vi "Initialize-buffers.vi"(8 "error in (no error)":errorcluster, 11 "Data ref. in":refnum<data-value>) -> (0 "error out":errorcluster, 3 "Data ref.":refnum<data-value>)   [LabVIEW 2013, in "CameraVision.lvlib" / "CV-Main.lvclass"]
uses:
  CV-Main.lvclass
  Buffers/CV-Buffers.lvclass
  CV-Main.lvclass/CV-Main.ctl
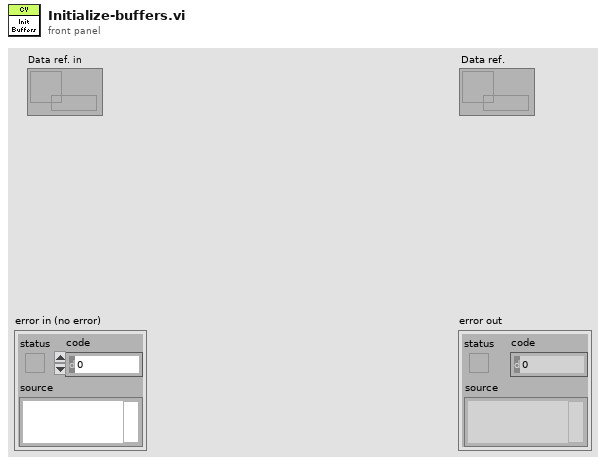
[diagram p1: front panel]
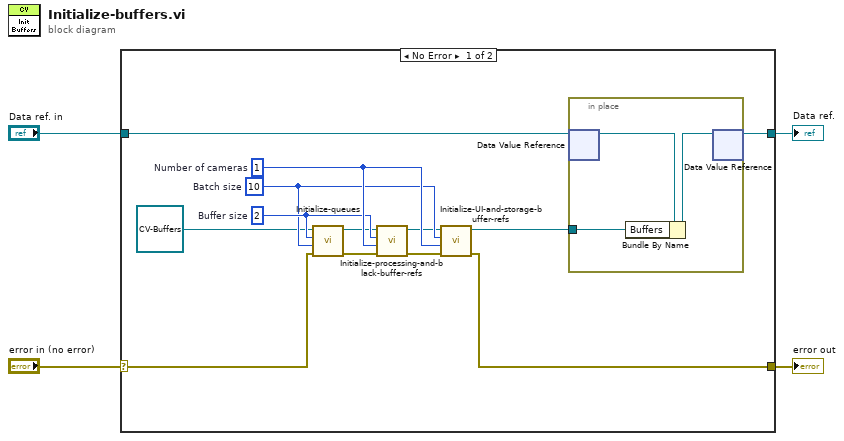
[diagram p0: block diagram]
diagram:
  n1 = case shown="No Error" "error in (no error)" {
    selector: "error in (no error)" -> [w12 w22]
    tunnel: [w5 w22] -> w3
    tunnel: "Data ref. in" -> [w17 w21]
    tunnel: [w16 w21] -> w1
    frame No Error {
      w14 = 2  # Buffer size
      w13 = 10  # Batch size
      w15 = 1  # Number of cameras
      n2 = call "Initialize-queues.vi"("error in (no error)"=w12, "Batch size"=w13, "Image buffer size"=w14, "Buffers in"=refnum<class "CV-Buffers.lvclass"> refnum) -> ("error out"=w11:errorcluster, "Buffers out"=w9:refnum<class "CV-Buffers.lvclass">)  [unwired: 6 in]
      n3 = call "Initialize-processing-and-black-buffer-refs.vi"("error in (no error)"=w11, "Number of cameras"=w15, "Image buffer size"=w14, "Buffers in"=w9) -> ("error out"=w10:errorcluster, "Buffers out"=w8:refnum<class "CV-Buffers.lvclass">)  [unwired: 6 in]
      n4 = call "Initialize-UI-and-storage-buffer-refs.vi"("error in (no error)"=w10, "Number of cameras"=w15, "Batch size"=w13, "Buffers in"=w8) -> ("error out"=w5:errorcluster, "Buffers out"=w6:refnum<class "CV-Buffers.lvclass">)  [unwired: 6 in]
      n5 = in-place {
        in-place-border: w6 -> [w18]
        n6 = in-place-dvr #1(w17) -> (w20:refnum<class "CV-Main.lvclass">)  [unwired: 1 out]
        n7 = Bundle By Name(cluster=w20, "Buffers"=w18) -> (w19:refnum<class "CV-Main.lvclass">)
        n8 = in-place-dvr #1(w19) -> (w16:refnum<data-value>)  [unwired: 1 out]
      }
    }
    frame Error {
    }
  }
  "error out" <- w3
  "Data ref." <- w1
